vi "cblas zgemv.vi"(0 "A":T3, 1 "x":cdb[](array[numeric]), 2 "y":cdb[](array[numeric]), 3 "alpha":cdb=1.0+0.0i, 4 "beta":cdb=1.0+0.0i, 5 "order":T1=101 items=["CblasRowMajor"=101, "CblasColMajor"=102], 6 "transA":T2=111 items=["CblasNoTrans"=111, "CblasTrans"=112, "CblasConjTrans "=113], 8 "lda":i32, 9 "m":i32=-1, 10 "incx":i32=1, 11 "n":i32=-1, 12 "incy":i32=1) -> (14 "zgemv":cdb[](array[numeric]), 19 "error":i32)   [LabVIEW 2017, in "NI_AALBLAS.lvlib"]
uses:
  <vilib>/Analysis/NI_AALBLAS.lvlib
  <vilib>/Analysis/Matrix/Datatypes/ComplexMatrix.ctl
  <vilib>/Analysis/BLAS.llb/Operation_Transpose.ctl
  <vilib>/Analysis/BLAS.llb/Order.ctl
  <resource>/lvblas.dll
  <vilib>/Analysis/Matrix/NI_Matrix.lvlib
panel:
  # "void cblas_zgemv(order, transA, m, n, *alpha, *A, lda, *x, incx, *beta, *y, incy)"
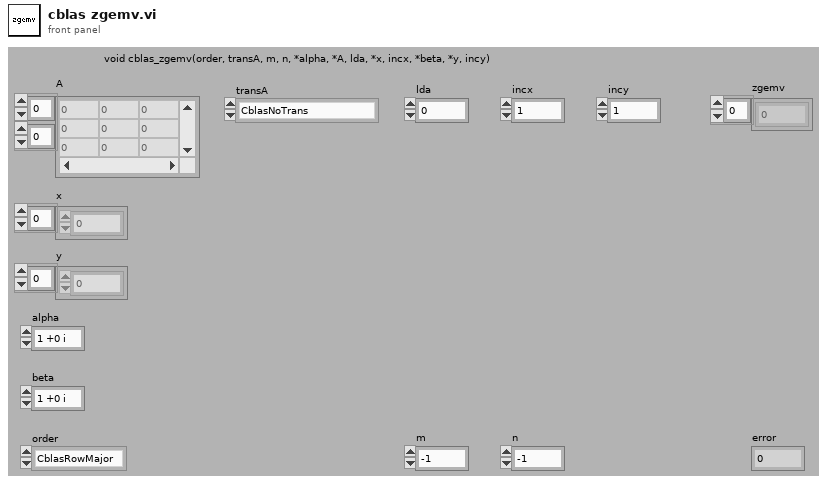
[diagram p1: front panel]
types:
  T1 = typedef "NI_AALBLAS.lvlib/Order.ctl" = i32
  T2 = typedef "NI_AALBLAS.lvlib/Operation_Transpose.ctl" = i32
  T3 = typedef "NI_Matrix.lvlib/ComplexMatrix.ctl" = cdb[][]
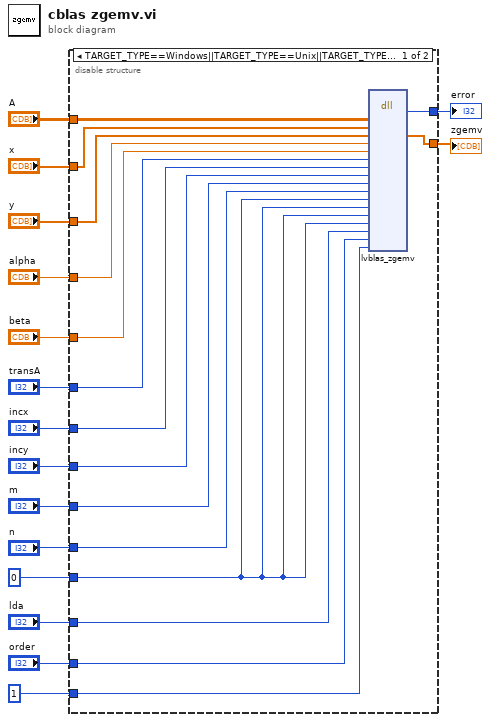
[diagram p0: block diagram]
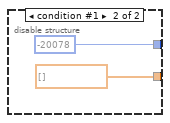
[diagram p2: hidden frame]
diagram:
  n1 = disable-structure shown="TARGET_TYPE==Windows||TARGET_TYPE==Unix||TARGET_TYPE==Mac||TARGET_TYPE==RT" {
    disable-tunnel: "x" -> [w32 _]
    disable-tunnel: "y" -> [w31 _]
    disable-tunnel: "alpha" -> [w30 _]
    disable-tunnel: [w29 cdb[] [] ("y")] -> w13
    disable-tunnel: "beta" -> [w28 _]
    disable-tunnel: "A" -> [w27 _]
    disable-tunnel: [w26 -20078 ("error")] -> w10
    disable-tunnel: "transA" -> [w25 _]
    disable-tunnel: 0 -> [w24 _]
    disable-tunnel: "lda" -> [w23 _]
    disable-tunnel: "order" -> [w22 _]
    disable-tunnel: "incx" -> [w20 _]
    disable-tunnel: "incy" -> [w21 _]
    disable-tunnel: "m" -> [w19 _]
    disable-tunnel: "n" -> [w18 _]
    disable-tunnel: 1 -> [w17 _]
    frame condition #0 (active) {
      n2 = dll-call lib="e:/builds/penguin/labview/branches/2017/dev/dist/resource/lvblas.*" fn="lvblas_zgemv" ("CBLAS.dll:CxMtrxxVectH")("a"=w27, "x"=w32, "y"=w31, "alpha"=w30, "beta"=w28, "OpA"=w25, "IncX"=w20, "IncY"=w21, "m"=w19, "n"=w18, "startARow"=w24, "startACol"=w24, "startX"=w24, "startY"=w24, "lda"=w23, "order"=w22, "check"=w17) -> ("error"=w26:i32, "y"=w29:cdb[])  [unwired: 19 in, 2 out]
    }
    frame condition #1 {
    }
  }
  "zgemv" <- w13
  "error" <- w10
